vi "VNS IRH3T Non Delay.vi"() -> ()   [LabVIEW 2013]
uses:
  Classes/OSSP_Problem.lvclass
  Classes/OSSP_Problem.lvclass/OSSP_Problem.ctl
  Classes/Scheduler_Class/Operation to Machine Job Tuple.vi
  GA/SubVIS/Remove Duplicates In Array.vi
  <vilib>/Analysis/NI_AALBase.lvlib
  <vilib>/Analysis/1siggen.llb/Riffle Array (I32).vi
  Classes/Scheduler.lvclass
panel:
  in  "Problem Type":enum16{"Taillard", "Brucker", "Gueret Prins"}(ring)
  in  "Instance Number for Taillard":dbl
  out "Tardiness(FIFO Engine)":u16
  out "VNS Result":u16[](array[numeric])
  out "Best Chromosome":i32[](array[numeric])
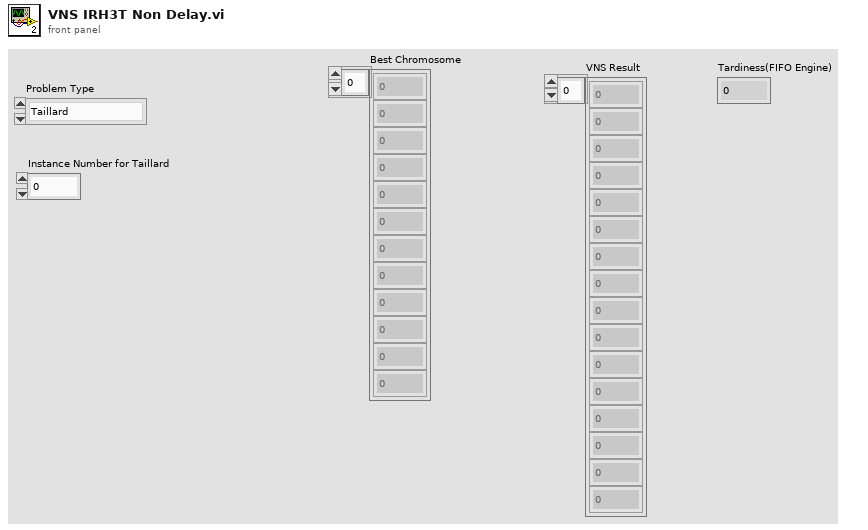
[diagram p1: front panel]
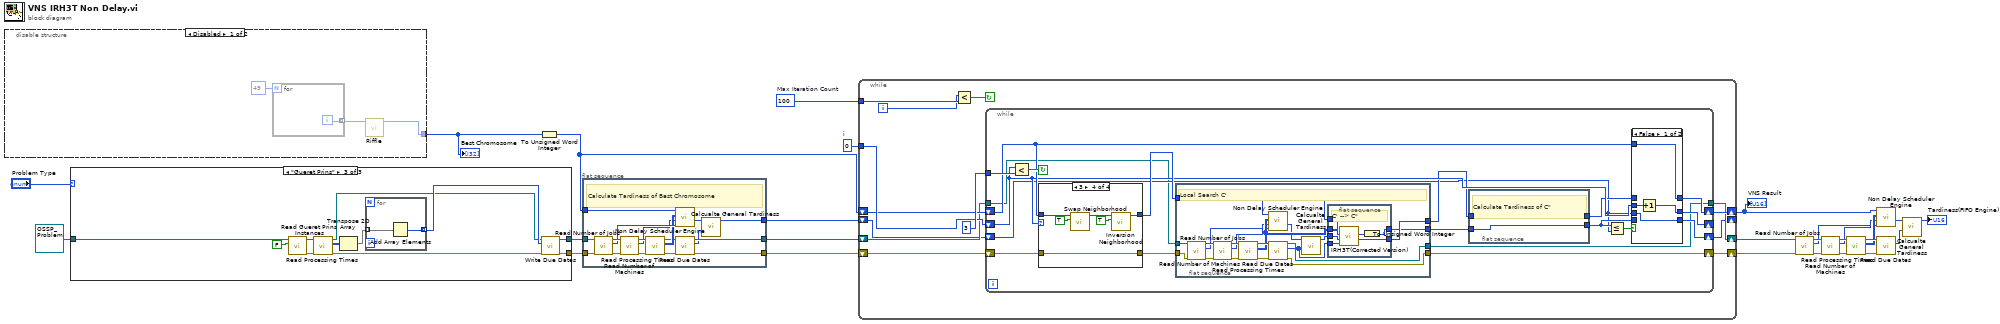
[diagram p0: block diagram]
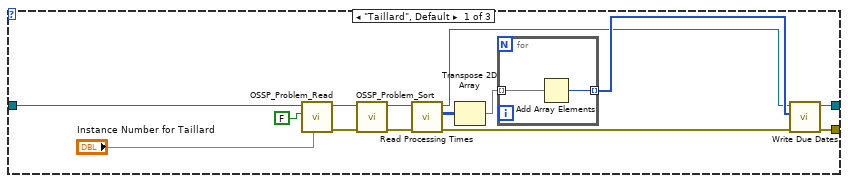
[diagram p2: hidden frame]
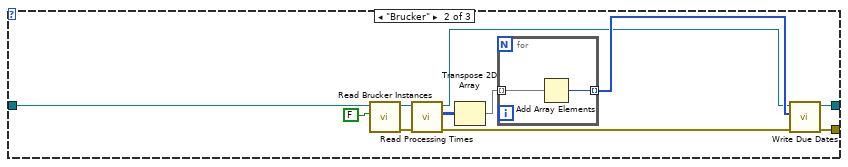
[diagram p3: hidden frame]
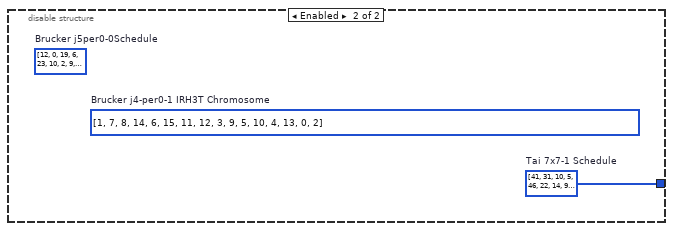
[diagram p4: hidden frame]
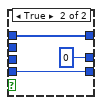
[diagram p5: hidden frame]
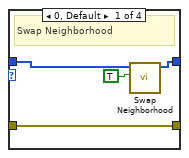
[diagram p6: hidden frame]
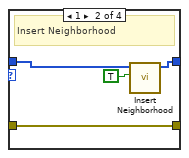
[diagram p7: hidden frame]
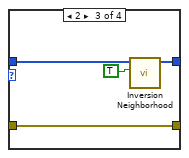
[diagram p8: hidden frame]
diagram:
  w25 = 0  # i
  w26 = 100  # Max Iteration Count
  n1 = disable-structure shown="Disabled" {
    disable-tunnel: [w27 w31] -> w24
    frame Disabled {
      n2 = for {
        N: 49 -> [_]
        tunnel: [w30] -> w28 mode=indexing
        i -> [w30]
      }
      n3 = call-poly <vilib>:"Riffle.vi"("X"=w28) -> ("Riffled {X}"=w27:i32[])  [unwired: 8 in, 2 out]
    }
    frame Enabled {
      w31 = i32[] [41, 31, 10, 5, 46, 22, 14, 9, 30, 39, 48, 21, 15, 3, 12, 34, 44, 32, 35, 27, 0, 38, 17, 36, 19, 8, 45, 37, 11, 29, 1, 28, 18, 16, 40, 23, 24, 13, 4, 43, 33, 7, 6, 25, 47, 2, 20, 42, 26]  # Tai 7x7-1 Schedule
      (unwired) i32[] [12, 0, 19, 6, 23, 10, 2, 9, 16, 8, 24, 11, 15, 7, 3, 20, 14, 18, 1, 5, 22, 13, 17, 21, 4]  # Brucker j5per0-0Schedule
      (unwired) i32[] [1, 7, 8, 14, 6, 15, 11, 12, 3, 9, 5, 10, 4, 13, 0, 2]  # Brucker j4-per0-1 IRH3T Chromosome
    }
  }
  "Best Chromosome" <- w24
  n4 = case shown="\"Gueret Prins\"" "Problem Type" {
    tunnel: refnum<class "OSSP_Problem.lvclass"> refnum ("OSSP_Problem.lvclass") -> [w45 w58 w71]
    tunnel: [w38 w53 w66] -> w21
    tunnel: [w37 w54 w67] -> w13
    frame "Taillard", Default {
      n5 = call "OSSP_Problem_Read.vi"("Instance Number"="Instance Number for Taillard", "Auto Mode"=FALSE, "OSSP_Problem.lvclass In"=w45) -> ("error out"=w42:errorcluster, "OSSP_Problem.lvclass Out"=w43:refnum<class "OSSP_Problem.lvclass">)  [unwired: 7 in]
      n6 = call "OSSP_Problem_Sort.vi"("error in (no error)"=w42, "OSSP_Problem.lvclass In"=w43) -> ("error out"=w40:errorcluster, "OSSP_Problem.lvclass Out"=w39:refnum<class "OSSP_Problem.lvclass">)  [unwired: 8 in]
      n7 = call "Read Processing Times.vi"("error in (no error)"=w40, "OSSP_Problem in"=w39) -> ("error out"=w32:errorcluster, "Processing Times"=w35:u16[][], "OSSP_Problem out"=w33:refnum<class "OSSP_Problem.lvclass">)  [unwired: 7 in]
      n8 = Transpose 2D Array(2D array=w35) -> (transposed array=w36:u16[][])
      n9 = for {
        tunnel: w36 -> [w47] mode=indexing
        tunnel: [w46] -> w34 mode=indexing
        n10 = Add Array Elements(numeric array=w47) -> (sum=w46:u16)
      }
      n11 = call "Write Due Dates.vi"("error in (no error)"=w32, "Due Dates"=w34, "OSSP_Problem in"=w33) -> ("error out"=w37:errorcluster, "OSSP_Problem out"=w38:refnum<class "OSSP_Problem.lvclass">)  [unwired: 7 in]
    }
    frame "Brucker" {
      n12 = call "Read Brucker Instances.vi"("Auto Mode"=FALSE, "OSSP_Problem in"=w58) -> ("error out"=w55:errorcluster, "OSSP_Problem out"=w56:refnum<class "OSSP_Problem.lvclass">)  [unwired: 8 in]
      n13 = call "Read Processing Times.vi"("error in (no error)"=w55, "OSSP_Problem in"=w56) -> ("error out"=w48:errorcluster, "Processing Times"=w51:u16[][], "OSSP_Problem out"=w49:refnum<class "OSSP_Problem.lvclass">)  [unwired: 7 in]
      n14 = Transpose 2D Array(2D array=w51) -> (transposed array=w52:u16[][])
      n15 = for {
        tunnel: w52 -> [w60] mode=indexing
        tunnel: [w59] -> w50 mode=indexing
        n16 = Add Array Elements(numeric array=w60) -> (sum=w59:u16)
      }
      n17 = call "Write Due Dates.vi"("error in (no error)"=w48, "Due Dates"=w50, "OSSP_Problem in"=w49) -> ("error out"=w54:errorcluster, "OSSP_Problem out"=w53:refnum<class "OSSP_Problem.lvclass">)  [unwired: 7 in]
    }
    frame "Gueret Prins" {
      n18 = call "Read Gueret Prins Instances.vi"("Auto Mode"=FALSE, "OSSP_Problem in"=w71) -> ("error out"=w68:errorcluster, "OSSP_Problem out"=w69:refnum<class "OSSP_Problem.lvclass">)  [unwired: 8 in]
      n19 = call "Read Processing Times.vi"("error in (no error)"=w68, "OSSP_Problem in"=w69) -> ("error out"=w61:errorcluster, "Processing Times"=w64:u16[][], "OSSP_Problem out"=w62:refnum<class "OSSP_Problem.lvclass">)  [unwired: 7 in]
      n20 = Transpose 2D Array(2D array=w64) -> (transposed array=w65:u16[][])
      n21 = for {
        tunnel: w65 -> [w73] mode=indexing
        tunnel: [w72] -> w63 mode=indexing
        n22 = Add Array Elements(numeric array=w73) -> (sum=w72:u16)
      }
      n23 = call "Write Due Dates.vi"("error in (no error)"=w61, "Due Dates"=w63, "OSSP_Problem in"=w62) -> ("error out"=w67:errorcluster, "OSSP_Problem out"=w66:refnum<class "OSSP_Problem.lvclass">)  [unwired: 7 in]
    }
  }
  n24 = To Unsigned Word Integer(number=w24) -> (unsigned 16bit integer=w20:u16[])
  n25 = flat-sequence {
    tunnel: w20 -> [w90]
    tunnel: [w74] -> w19
    tunnel: w21 -> [w89]
    tunnel: [w83] -> w18
    tunnel: w13 -> [w82]
    tunnel: [w78] -> w12
    frame #0 {
      # "Calculate Tardiness of Best Chromosome"
      n26 = call "Read Number of Jobs.vi"("error in (no error)"=w82, "OSSP_Problem in"=w89) -> ("error out"=w81:errorcluster, "Number of Jobs"=w87:i32, "OSSP_Problem out"=w88:refnum<class "OSSP_Problem.lvclass">)  [unwired: 7 in]
      n27 = call "Read Number of Machines.vi"("error in (no error)"=w81, "OSSP_Problem in"=w88) -> ("error out"=w80:errorcluster, "Number of Machines"=w77:i32, "OSSP_Problem out"=w86:refnum<class "OSSP_Problem.lvclass">)  [unwired: 7 in]
      n28 = call "Read Processing Times.vi"("error in (no error)"=w80, "OSSP_Problem in"=w86) -> ("error out"=w79:errorcluster, "Processing Times"=w85:u16[][], "OSSP_Problem out"=w84:refnum<class "OSSP_Problem.lvclass">)  [unwired: 7 in]
      n29 = call "Non Delay Scheduler Engine.vi"("Number of  Jobs"=w87, "Number of Machines"=w77, "Processing Times"=w85, "Schedule"=w90) -> ("Job Completion Times"=w76:u16[])  [unwired: 2 in, 5 out]
      n30 = call "Read Due Dates.vi"("error in (no error)"=w79, "OSSP_Problem in"=w84) -> ("error out"=w78:errorcluster, "Due Dates"=w75:u16[], "OSSP_Problem out"=w83:refnum<class "OSSP_Problem.lvclass">)  [unwired: 7 in]
      n31 = call "Calcualte General Tardiness.vi"("Due Dates"=w75, "Job Completion Times"=w76) -> ("Total Tardiness (U16)"=w74:u16)  [unwired: 9 in]
    }
  }
  n32 = while {
    tunnel: w26 -> [w103]
    tunnel: w25 -> [w100]
    shift-right: [w98] -> w7
    shift-left: w20 -> [w97]
    shift-right: [w96] -> w17
    shift-left: w18 -> [w95]
    shift-right: [w94] -> _
    shift-left: w19 -> [w93]
    shift-right: [w91] -> w11
    shift-left: w12 -> [w92]
    i -> [w99]
    stop <- w102 continue-if-true
    n33 = Less?(x=w99, y=w103) -> (x < y?=w102:bool)
    n34 = while {
      tunnel: 3 -> [w119]
      shift-right: [w118] -> _
      shift-left: w100 -> [w115]
      shift-right: [w117] -> w98
      shift-left: w97 -> [w116]
      shift-right: [w110] -> w94
      shift-left: w93 -> [w109]
      tunnel: w95 -> [w108]
      tunnel: [w107] -> w96
      shift-right: [w104] -> w91
      shift-left: w92 -> [w106]
      stop <- w122 continue-if-true
      n35 = Less?(x=w115, y=w119) -> (x < y?=w122:bool)
      n36 = case shown="3" w115 {
        tunnel: w116 -> [w161 w165 w169 w175]
        tunnel: [w160 w164 w168 w173] -> w121
        tunnel: w106 -> [w158 w162 w166 w170]
        tunnel: [w158 w162 w166 w170] -> w105
        frame 0, Default {
          # "Swap Neighborhood"
          n37 = call "Swap Neighborhood.vi"("Generate Random Indices?"=TRUE, "Schedule In"=w161) -> ("Schedule Out"=w160:u16[])  [unwired: 9 in]
        }
        frame 1 {
          # "Insert Neighborhood"
          n38 = call "Insert Neighborhood.vi"("Generate Random Indices?"=TRUE, "C'"=w165) -> ("Chromosome Out"=w164:u16[])  [unwired: 9 in]
        }
        frame 2 {
          n39 = call "Inversion Neighborhood.vi"("Generate Random Indices?"=TRUE, "Schedule in"=w169) -> ("Schedule out"=w168:u16[])  [unwired: 9 in]
        }
        frame 3 {
          n40 = call "Swap Neighborhood.vi"("Generate Random Indices?"=TRUE, "Schedule In"=w175) -> ("Schedule Out"=w174:u16[])  [unwired: 9 in]
          n41 = call "Inversion Neighborhood.vi"("Generate Random Indices?"=TRUE, "Schedule in"=w174) -> ("Schedule out"=w173:u16[])  [unwired: 9 in]
        }
      }
      n42 = flat-sequence {
        tunnel: w121 -> [w138]
        tunnel: [w150] -> w113
        tunnel: [w149] -> w114
        tunnel: w108 -> [w148]
        tunnel: [w144] -> w107
        tunnel: w105 -> [w143]
        tunnel: [w139] -> w104
        frame #0 {
          # "Local Search C'"
          n43 = call "Read Number of Jobs.vi"("error in (no error)"=w143, "OSSP_Problem in"=w148) -> ("error out"=w142:errorcluster, "Number of Jobs"=w135:i32, "OSSP_Problem out"=w147:refnum<class "OSSP_Problem.lvclass">)  [unwired: 7 in]
          n44 = call "Read Number of Machines.vi"("error in (no error)"=w142, "OSSP_Problem in"=w147) -> ("error out"=w141:errorcluster, "Number of Machines"=w136:i32, "OSSP_Problem out"=w146:refnum<class "OSSP_Problem.lvclass">)  [unwired: 7 in]
          n45 = call "Read Processing Times.vi"("error in (no error)"=w141, "OSSP_Problem in"=w146) -> ("error out"=w140:errorcluster, "Processing Times"=w137:u16[][], "OSSP_Problem out"=w145:refnum<class "OSSP_Problem.lvclass">)  [unwired: 7 in]
          n46 = call "Non Delay Scheduler Engine.vi"("Number of  Jobs"=w135, "Number of Machines"=w136, "Processing Times"=w137, "Schedule"=w138) -> ("Job Completion Times"=w134:u16[])  [unwired: 2 in, 5 out]
          n47 = call "Read Due Dates.vi"("error in (no error)"=w140, "OSSP_Problem in"=w145) -> ("error out"=w139:errorcluster, "Due Dates"=w133:u16[], "OSSP_Problem out"=w144:refnum<class "OSSP_Problem.lvclass">)  [unwired: 7 in]
          n48 = call "Calcualte General Tardiness.vi"("Due Dates"=w133, "Job Completion Times"=w134) -> ("Total Tardiness (U16)"=w132:u16)  [unwired: 9 in]
          n49 = flat-sequence {
            tunnel: w138 -> [w157]
            tunnel: [w151] -> w150
            tunnel: w137 -> [w156]
            tunnel: w133 -> [w155]
            tunnel: [w153] -> w149
            tunnel: w132 -> [w152]
            frame #0 {
              # "C' --> C\""
              n50 = call "IRH3T(Corrected Version).vi"("Due Dates"=w155, "Initial Tardiness"=w152, "Schedule 2B Improved"=w157, "Proocessing Times  (Machines x Jobs)"=w156) -> ("IRH3T Schedule Out"=w151:u16[], "Total Tardiness"=w154:u16)  [unwired: 5 in, 1 out]
              n51 = To Unsigned Word Integer(number=w154) -> (unsigned 16bit integer=w153:u16)
            }
          }
        }
      }
      n52 = flat-sequence {
        tunnel: w113 -> [w123]
        tunnel: [w124] -> w111
        tunnel: w114 -> [w124]
        tunnel: [w123] -> w112
        frame #0 {
          # "Calculate Tardiness of C\""
        }
      }
      n53 = Less Or Equal?(x=w111, y=w109) -> (x <= y?=w120:bool)
      n54 = case shown="False" w120 {
        tunnel: w115 -> [w127 _]
        tunnel: w112 -> [_ w130]
        tunnel: [w128 0] -> w118
        tunnel: [w126 w130] -> w117
        tunnel: w116 -> [w126 _]
        tunnel: w111 -> [_ w129]
        tunnel: [w125 w129] -> w110
        tunnel: w109 -> [w125 _]
        frame False {
          n55 = Increment(x=w127) -> (x+1=w128:i32)
        }
        frame True {
        }
      }
    }
  }
  "VNS Result" <- w7
  n56 = call "Read Number of Jobs.vi"("error in (no error)"=w11, "OSSP_Problem in"=w17) -> ("error out"=w10:errorcluster, "Number of Jobs"=w4:i32, "OSSP_Problem out"=w16:refnum<class "OSSP_Problem.lvclass">)  [unwired: 7 in]
  n57 = call "Read Number of Machines.vi"("error in (no error)"=w10, "OSSP_Problem in"=w16) -> ("error out"=w9:errorcluster, "Number of Machines"=w5:i32, "OSSP_Problem out"=w15:refnum<class "OSSP_Problem.lvclass">)  [unwired: 7 in]
  n58 = call "Read Processing Times.vi"("error in (no error)"=w9, "OSSP_Problem in"=w15) -> ("error out"=w8:errorcluster, "Processing Times"=w6:u16[][], "OSSP_Problem out"=w14:refnum<class "OSSP_Problem.lvclass">)  [unwired: 7 in]
  n59 = call "Non Delay Scheduler Engine.vi"("Number of  Jobs"=w4, "Number of Machines"=w5, "Processing Times"=w6, "Schedule"=w7) -> ("Job Completion Times"=w3:u16[])  [unwired: 2 in, 5 out]
  n60 = call "Read Due Dates.vi"("error in (no error)"=w8, "OSSP_Problem in"=w14) -> ("Due Dates"=w2:u16[])  [unwired: 7 in, 2 out]
  n61 = call "Calcualte General Tardiness.vi"("Due Dates"=w2, "Job Completion Times"=w3) -> ("Total Tardiness (U16)"=→"Tardiness(FIFO Engine)":u16)  [unwired: 9 in]
